vi "Close.vi"(8 "error in":errorcluster, 11 "Power Supply in":refnum<class "Power Supply.lvclass">) -> (0 "error out":errorcluster, 3 "Power Supply out":refnum<class "Power Supply.lvclass">)   [LabVIEW 2023, in "Power Supply.lvclass"]
uses:
  Power Supply.lvclass
  Power Supply.lvclass/Power Supply.ctl
  <vilib>/ADAS Replay HIL/AdasHilServices/AdasHilServices Fill In Error Info Ex.vi
  <vilib>/ADAS Replay HIL/AdasHilServices/AdasHilChannelServices.lvlib
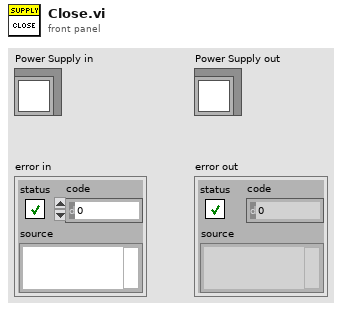
[diagram p1: front panel]
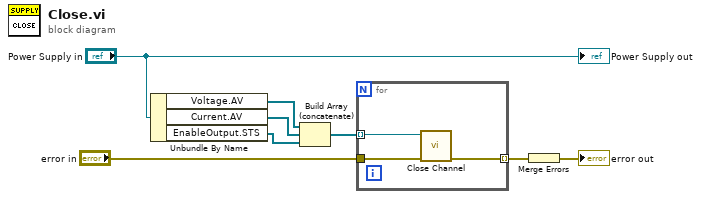
[diagram p0: block diagram]
diagram:
  n1 = Unbundle By Name("Power Supply in") -> ("Voltage.AV"=w7:refnum<k21>[], "Current.AV"=w6:refnum<k21>[], "EnableOutput.STS"=w5:refnum<k21>[])
  n2 = Build Array (concatenate)(w7, w6, w5) -> (w4:refnum<k21>[])
  n3 = for {
    tunnel: w4 -> [w11] mode=indexing
    tunnel: "error in" -> [w10]
    tunnel: [w9] -> w2 mode=indexing
    n4 = call <vilib>:"Close Channel.vi"("error in"=w10, "ADAS HIL Channel"=w11) -> ("error out"=w9:errorcluster)  [unwired: 9 in]
  }
  n5 = Merge Errors(w2) -> (→"error out":errorcluster)
  "Power Supply out" <- "Power Supply in"
